vi "from string.vi"(8 "error in":errorcluster, 9 "data":string, 10 "version":string, 11 "System configuration in":refnum<class "System configuration.lvclass">) -> (0 "error out":errorcluster, 3 "System configuration out":refnum<class "System configuration.lvclass">)   [LabVIEW 2025, in "System.lvlib" / "System configuration.lvclass"]
doc: "Provides an interface for loading a module configuration from a file or other serialized data source. It is recommended that all children of this class store data in two sets--data required for its own initialization, and any data required for parent initialization--and that each implementation uses the <b>Call Parent Method</b> primitive to de-serialize parent information.Copyright 2017 National Instruments Corporation\n\nLicensed under the Apache License, Version 2.0 (the \"License\"); you may not use this file except in compliance with the License. You may obtain a copy of the License at http://www.apache.org/licenses/LICENSE-2.0\nUnless required by applicable law or agreed to in writing, software distributed under the License is distributed on an \"AS IS\" BASIS, WITHOUT WARRANTIES OR CONDITIONS OF ANY KIND, either express or implied. See the License for the specific language governing permissions and limitations under the License."
uses:
  System configuration.lvclass
  System configuration.lvclass/System configuration.ctl
  Users/Public/Documents/Sandia National Labs/TSS Plugin/CEF.lvlibp/serializable configuration/CEF_serializable configuration.lvclass
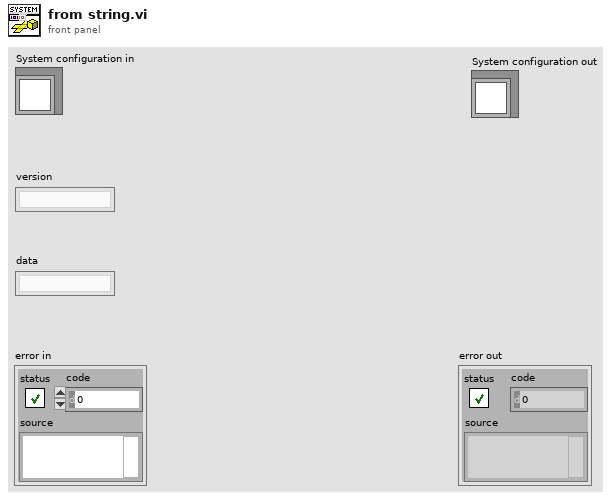
[diagram p1: front panel]
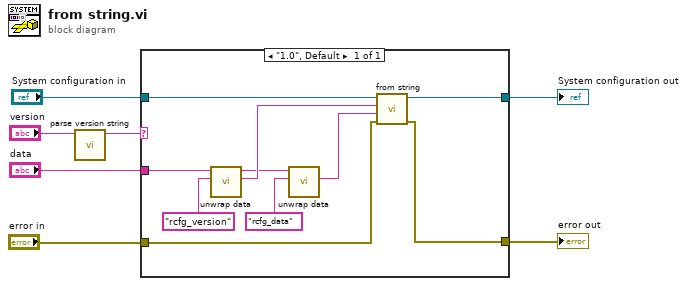
[diagram p0: block diagram]
diagram:
  n1 = call "parse version string.vi"("full version"="version") -> ("major.minor version"=w4:string)  [unwired: 7 in, 3 out]
  n2 = case shown="\"1.0\", Default" w4 {
    tunnel: "System configuration in" -> [w17]
    tunnel: [w16] -> w2
    tunnel: "data" -> [w15]
    tunnel: "error in" -> [w10]
    tunnel: [w9] -> w1
    frame "1.0", Default {
      n3 = call "unwrap data.vi"("identifier"="rcfg_version" ("additional identifier"), "data to unwrap"=w15) -> ("unwrapped data"=w13:string, "remaining string"=w12:string)  [unwired: 8 in]
      n4 = call "unwrap data.vi"("identifier"="rcfg_data" ("additional identifier"), "data to unwrap"=w12) -> ("unwrapped data"=w8:string)  [unwired: 8 in, 1 out]
      n5 = call-parent "from string.vi"("error in"=w10, "data"=w8, "version"=w13, "CEF_Configuration in"=w17) -> ("error out"=w9:errorcluster, "CEF_Configuration out"=w16:refnum<class "System configuration.lvclass">)  [unwired: 6 in]
    }
  }
  "error out" <- w1
  "System configuration out" <- w2
